vi "获取用户列表.vi"(8 "error in (no error)":errorcluster, 11 "数据库连接引用":T2) -> (0 "职类分段索引":i32[](array[numeric]), 1 "未绑定":string[][](array[string]), 2 "已绑定":string[][](array[string]), 3 "用户列表":string[][](array[string]), 4 "列名（参考）":T1(ring), 6 "error out":errorcluster)   [LabVIEW 2013, in "数据库操作.lvclass"]
uses:
  <vilib>/addons/database/Connection.llb/Conn ObjectReference.ctl
  <vilib>/addons/database/NI_Database_API.lvlib
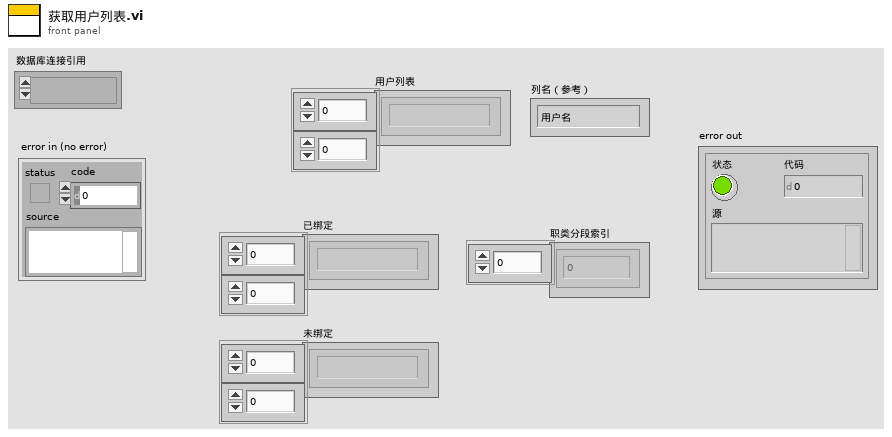
[diagram p1: front panel]
types:
  T1 = enum16{"用户名", "设备MAC", "设备状态", "密码", "职类", "姓名", "电话", "邮箱", "备注", "最后活动"}
  T2 = typedef "NI_Database_API.lvlib/Conn ObjectReference.ctl" = refnum<k1>
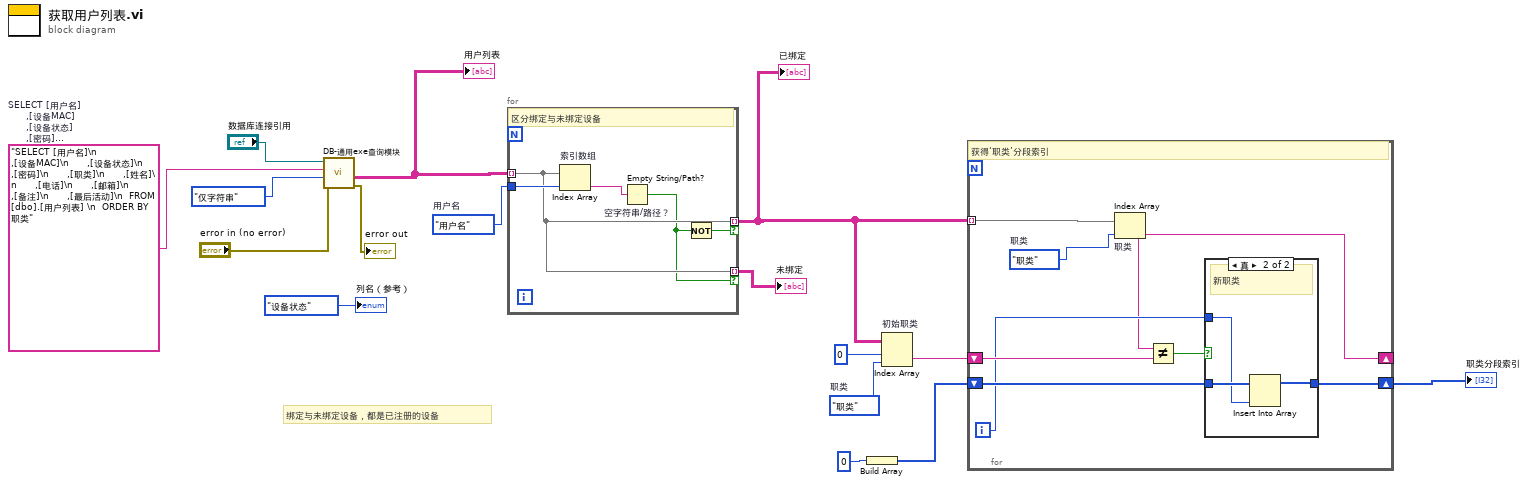
[diagram p0: block diagram]
diagram:
  w8 = T1."职类"  # 职类
  w11 = T1."用户名"  # 用户名
  w16 = "SELECT [用户名]\n      ,[设备MAC]\n      ,[设备状态]\n      ,[密码]\n      ,[职类]\n      ,[姓名]\n      ,[电话]\n      ,[邮箱]\n      ,[备注]\n      ,[最后活动]\n  FROM [dbo].[用户列表] \n  ORDER BY 职类"  # SELECT [用户名]       ,[设备MAC]       ,[设备状态]       ,[密码]       ,[职类]       ,[姓名]       ,[电话]       ,[邮箱]       ,[备注]       ,[最后活动]   FROM [dbo].[用户列表]    ORDER BY 职类
  # "绑定与未绑定设备，都是已注册的设备"
  n1 = call "DB-通用exe查询模块.vi"("error in (no error)"="error in (no error)", "解析模式"=enum16{"仅数值", "仅字符串", "数值与字符串"}."仅字符串", "SQL query"=w16, "数据库连接引用"="数据库连接引用") -> ("error out"=→"error out":errorcluster, "字符串数据"=w12:string[][])  [unwired: 4 in, 2 out]
  "用户列表" <- w12
  n2 = for {
    tunnel: w12 -> [w19] mode=indexing
    tunnel: w11 -> [w21]
    tunnel: [w19] -> w4 mode=indexing if=w17
    tunnel: [w19] -> w10 mode=indexing if=w18
    # "区分绑定与未绑定设备"
    n3 = Index Array "索引数组"(array=w19, index=w21) -> (element=w20:string)
    n4 = Empty String/Path? "空字符串/路径？"(string/path=w20) -> (empty?=w18:bool)
    n5 = Not(x=w18) -> (.not. x?=w17:bool)
  }
  "已绑定" <- w4
  "未绑定" <- w10
  n6 = Build Array(0) -> (w5:i32[])
  n7 = Index Array "初始职类"(array=w4, index (row)=0, index (col)=w8) -> (element=w7:string)
  n8 = for {
    tunnel: w4 -> [w28] mode=indexing
    shift-right: [w23] -> _
    shift-left: w7 -> [w29]
    shift-right: [w25] -> w3
    shift-left: w5 -> [w27]
    i -> [w24]
    w22 = T1."职类"  # 职类
    # "获得‘职类’分段索引"
    n9 = Index Array "职类"(array=w28, index=w22) -> (element=w23:string)
    n10 = Not Equal?(x=w23, y=w29) -> (x != y?=w26:bool)
    n11 = case shown="真" w26 {
      tunnel: w27 -> [w30 w33]
      tunnel: w24 -> [_ w32]
      tunnel: [w30 w31] -> w25
      frame False {
        # "同职类"
      }
      frame True {
        # "新职类"
        n12 = Insert Into Array(array=w33, new element=w32) -> (w31:i32[])  [unwired: 1 in]
      }
    }
  }
  "职类分段索引" <- w3
  "列名（参考）" <- T1."设备状态"
